vi "CoboltLaser_LEDstatusGet.vi"(0 "ComPort":refnum<visa-resource-name>, 3 "CheckResponse":bool=TRUE, 7 "error in (no error)":errorcluster) -> (20 "ComPortOut":refnum<visa-resource-name>, 21 "PowerOn":bool, 22 "LaserOn":bool, 23 "LaserLock":bool, 24 "Error":bool, 27 "error out":errorcluster)   [LabVIEW 2019]
doc: "Use this template to build a VI to use as a subVI."
panel:
  out "ResponseOK":bool
  out "Response":string
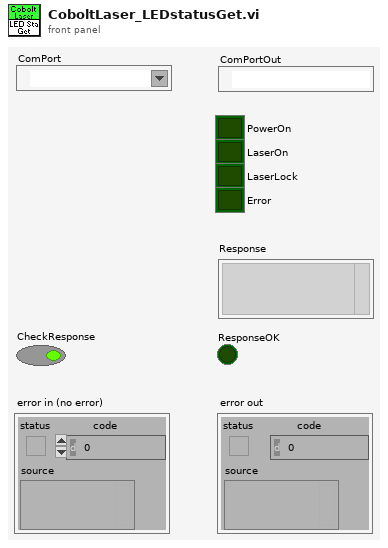
[diagram p1: front panel]
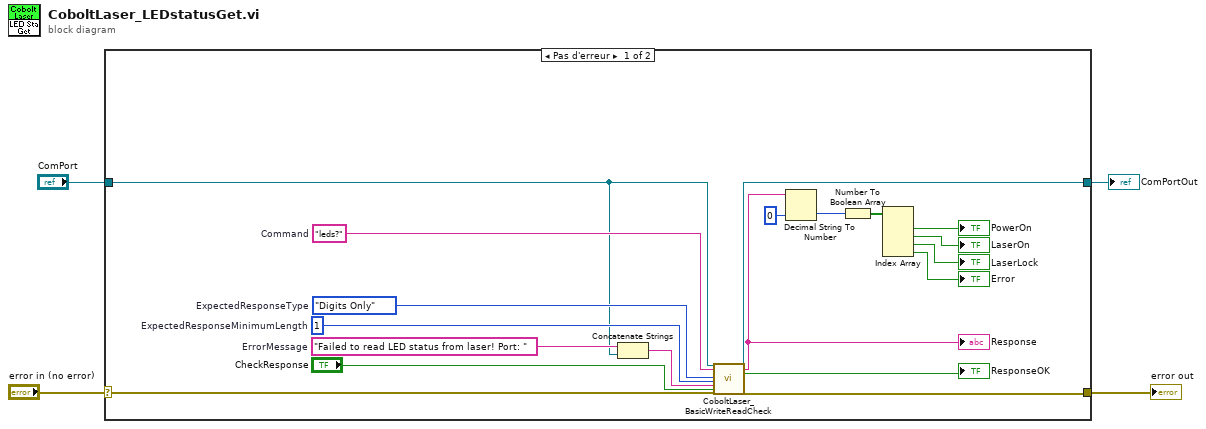
[diagram p0: block diagram]
diagram:
  n1 = case shown="Pas d'erreur" "error in (no error)" {
    selector: "error in (no error)" -> [w23 w25]
    tunnel: [w22 w25] -> w3
    tunnel: "ComPort" -> [w6 w24]
    tunnel: [w5 w24] -> w1
    frame No Error {
      w19 = 1  # ExpectedResponseMinimumLength
      w20 = enum16{"Any", "Digits Only", "Non-Digits Only"}."Digits Only"  # ExpectedResponseType
      w16 = "Failed to read LED status from laser! Port: "  # ErrorMessage
      w21 = "leds?"  # Command
      n2 = Concatenate Strings(w16, w6) -> (w15:string)
      n3 = call <userlib>:"CoboltLaser_BasicWriteReadCheck.vi"("ComPort"=w6, "Command"=w21, "ExpectedResponseType"=w20, "ExpectedResponseMinimumLength"=w19, "ErrorMessage"=w15, "GenerateError"="CheckResponse", "error in (no error)"=w23) -> ("ComPortOut"=w5:refnum<visa-resource-name>, "Response"=w14:string, "ResponseOK"=→"ResponseOK":bool, "error out"=w22:errorcluster)  [unwired: 17 in]
      "Response" <- w14
      n4 = Decimal String To Number(string=w14, default (0L)=i16 0 ("default (0 I32)")) -> (number=w13:i16)  [unwired: 1 in, 1 out]
      n5 = Number To Boolean Array(number=w13) -> (Boolean array=w11:bool[])
      n6 = Index Array(array=w11) -> (element #1=→"PowerOn":bool, element #2=→"LaserOn":bool, element #3=→"LaserLock":bool, element #4=→"Error":bool)  [unwired: 4 in]
    }
    frame Error {
    }
  }
  "error out" <- w3
  "ComPortOut" <- w1
